vi "state-cluster_test.vi"() -> ()   [LabVIEW 2024]
panel:
  out "remaining queue":T1(array[cluster])
  out "heartbeat":bool
  out "deleted portion":T2
  in  "stop":bool
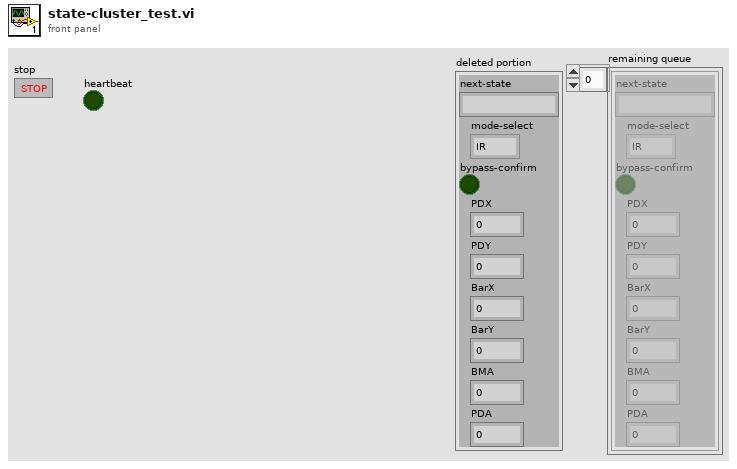
[diagram p1: front panel]
types:
  T1 = cluster{"next-state":string, "mode-select":enum32{"IR", "Pure", "Bulk", "Bar Out", "custom"}, "bypass-confirm":bool, "PDX":dbl, "PDY":dbl, "BarX":dbl, "BarY":dbl, "BMA":dbl, "PDA":dbl}[]
  T2 = cluster{"next-state":string, "mode-select":enum32{"IR", "Pure", "Bulk", "Bar Out", "custom"}, "bypass-confirm":bool, "PDX":dbl, "PDY":dbl, "BarX":dbl, "BarY":dbl, "BMA":dbl, "PDA":dbl}
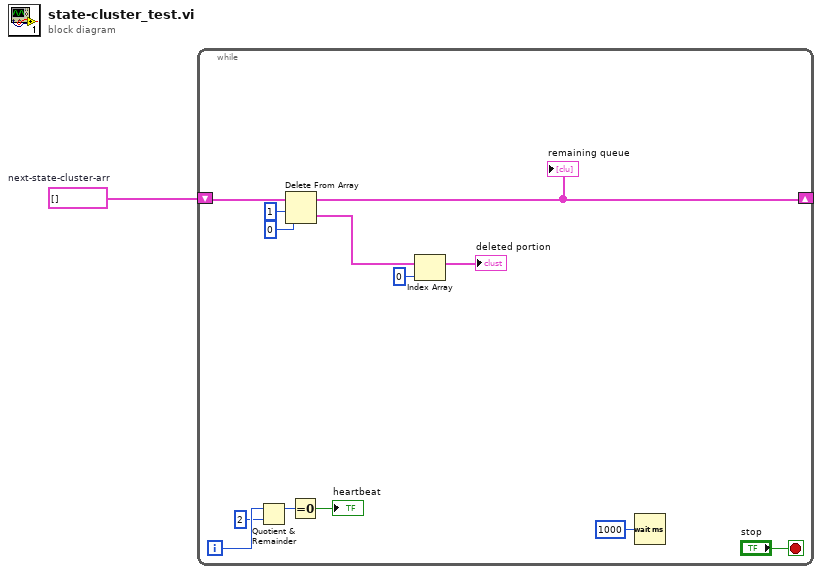
[diagram p0: block diagram]
diagram:
  w1 = T1 []  # next-state-cluster-arr
  n1 = while {
    shift-right: [w9] -> _
    shift-left: w1 -> [w12]
    i -> [w7]
    stop <- "stop" stop-if-true
    n2 = Quotient & Remainder(x=w7, y=2) -> (x-y*floor(x/y)=w5:i32)  [unwired: 1 out]
    n3 = Delete From Array(array=w12, length=1, index=0) -> (deleted portion=w8:T1, array with subset deleted=w9:T1)
    "remaining queue" <- w9
    n4 = Equal To 0?(x=w5) -> (x = 0?=→"heartbeat":bool)
    n5 = Index Array(array=w8, index=0) -> (element=→"deleted portion":T2)
    n6 = Wait (ms)(milliseconds to wait=u32 1000) -> ()  [unwired: 1 out]
  }
